vi "Create PPL Migrator.vi"(0 "Project Refnum":refnum<vi>, 5 "Plug-in name":string, 7 "Main VI Name":string, 9 "Library name":string, 11 "error in (no error)":errorcluster) -> (4 "project ref out":refnum<vi>, 6 "path":path, 15 "error out":errorcluster)   [LabVIEW 2021, in "NI_AB_API_PPL_Extensions.lvclass"]
uses:
  NI_AB_API_PPL_Extensions.lvclass
  InstrumentStudio Plug-In Editor.lvlib
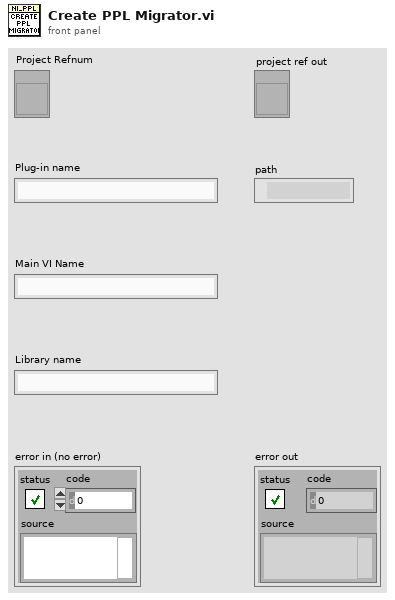
[diagram p1: front panel]
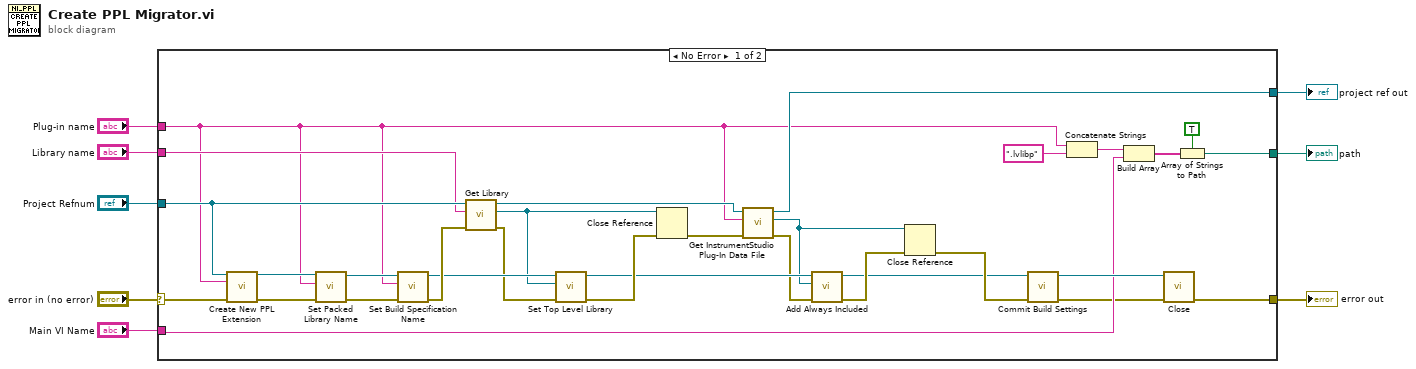
[diagram p0: block diagram]
diagram:
  n1 = case shown="No Error" "error in (no error)" {
    selector: "error in (no error)" -> [w39 w40]
    tunnel: "Project Refnum" -> [w38 w41]
    tunnel: "Plug-in name" -> [w11 _]
    tunnel: [w22 w41] -> w6
    tunnel: [w27 _] -> w5
    tunnel: "Library name" -> [w14 _]
    tunnel: "Main VI Name" -> [w13 _]
    tunnel: [w9 w40] -> w3
    frame No Error {
      n2 = call "Create New PPL Extension.vi"("Project Refnum"=w38, "Build specification name"=w11, "error in (no error)"=w39) -> ("NI_AB_API_Build out"=w12:refnum<class "NI_AB_API_PPL_Extensions.lvclass">, "error out"=w24:errorcluster)  [unwired: 11 in]
      n3 = call-dynamic "Set Packed Library Name.vi"("error in (no error)"=w24, "Packed library name"=w11, "PPL in"=w12) -> ("error out"=w25:errorcluster, "PPL out"=w26:refnum<class "NI_AB_API_PPL_Extensions.lvclass">)  [unwired: 7 in]
      n4 = call-dynamic "Set Build Specification Name.vi"("error in (no error)"=w25, "Build Specification Name"=w11, "NI_AB_API_PPL in"=w26) -> ("error out"=w37:errorcluster, "NI_AB_API_PPL out"=w36:refnum<class "NI_AB_API_PPL_Extensions.lvclass">)  [unwired: 7 in]
      n5 = call "Get Library.vi"("error in"=w37, "library name"=w14, "project ref"=w38) -> ("error out"=w35:errorcluster, "library item"=w30:refnum<vi>, "project ref out"=w23:refnum<vi>)  [unwired: 5 in, 1 out]
      n6 = call-dynamic "Set Top Level Library.vi"("error in (no error)"=w35, "ProjectItem Refnum"=w30, "PPL in"=w36) -> ("error out"=w34:errorcluster, "PPL out"=w21:refnum<class "NI_AB_API_PPL_Extensions.lvclass">)  [unwired: 7 in]
      n7 = Close Reference(reference=w30, error in (no error)=w34) -> (error out=w15:errorcluster)
      n8 = call "Get InstrumentStudio Plug-In Data File.vi"("error in"=w15, "library name"=w11, "project ref"=w23) -> ("error out"=w16:errorcluster, "Document item"=w20:refnum<vi>, "project ref out"=w22:refnum<vi>)  [unwired: 5 in, 1 out]
      n9 = call-dynamic "Add Always Included.vi"("error in (no error)"=w16, "ProjectItem Refnum"=w20, "PPL in"=w21) -> ("error out"=w19:errorcluster, "PPL out"=w17:refnum<class "NI_AB_API_PPL_Extensions.lvclass">)  [unwired: 7 in]
      n10 = Close Reference(reference=w20, error in (no error)=w19) -> (error out=w18:errorcluster)
      n11 = call-dynamic "Commit Build Settings.vi"("error in (no error)"=w18, "PPL in"=w17) -> ("error out"=w10:errorcluster, "PPL out"=w31:refnum<class "NI_AB_API_PPL_Extensions.lvclass">)  [unwired: 8 in]
      n12 = Concatenate Strings(w11, ".lvlibp" ("string")) -> (w32:string)
      n13 = Build Array(w32, w13) -> (w28:string[])
      n14 = call-dynamic "Close.vi"("error in (no error)"=w10, "DLL in"=w31) -> ("error out"=w9:errorcluster)  [unwired: 9 in]
      n15 = Array of Strings to Path(0:w28, 1:TRUE ("relative")) -> (2:w27:path)
    }
    frame Error {
    }
  }
  "error out" <- w3
  "project ref out" <- w6
  "path" <- w5
